vi "Create Device Tree.vi"(8 "error in (no error)":errorcluster caption="错误输入（无错误）", 9 "Item Indent":i16 caption="项缩进", 10 "Tree Control Ref":refnum<vi> caption="树形控件引用", 11 "Project Item Array":refnum<vi>[](array[refnum]) caption="项目项集合") -> (0 "error out":errorcluster caption="错误输出")   [LabVIEW 2013]
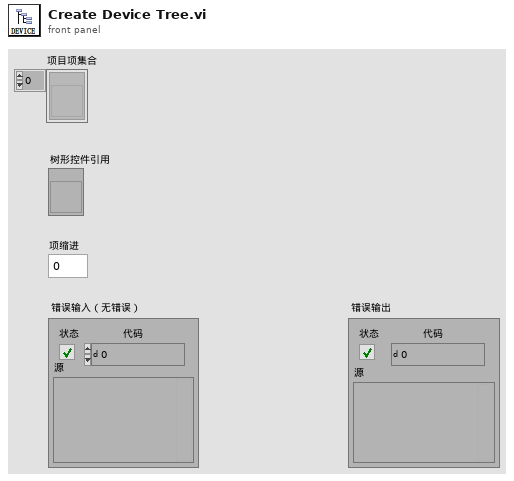
[diagram p1: front panel]
types:
  T1 = cluster{"Left Cell String":string, "Child Text":string[], "Child Tag":string, "Item Indent":i32, "Child Only?":bool, "Glyph Index":i32}
  T2 = typedef "imagedata.ctl" = cluster{"image type":i32, "image depth":i32, "image":u8[], "mask":u8[], "colors":u32[], "Rectangle":cluster{"left":i16, "top":i16, "right":i16, "bottom":i16}}
  T3 = cluster{"Left Cell String":string, "Child Text":string[], "Child Tag":string, "Item Indent":i32, "Child Only?":bool, "Glyph Index":i32}[]
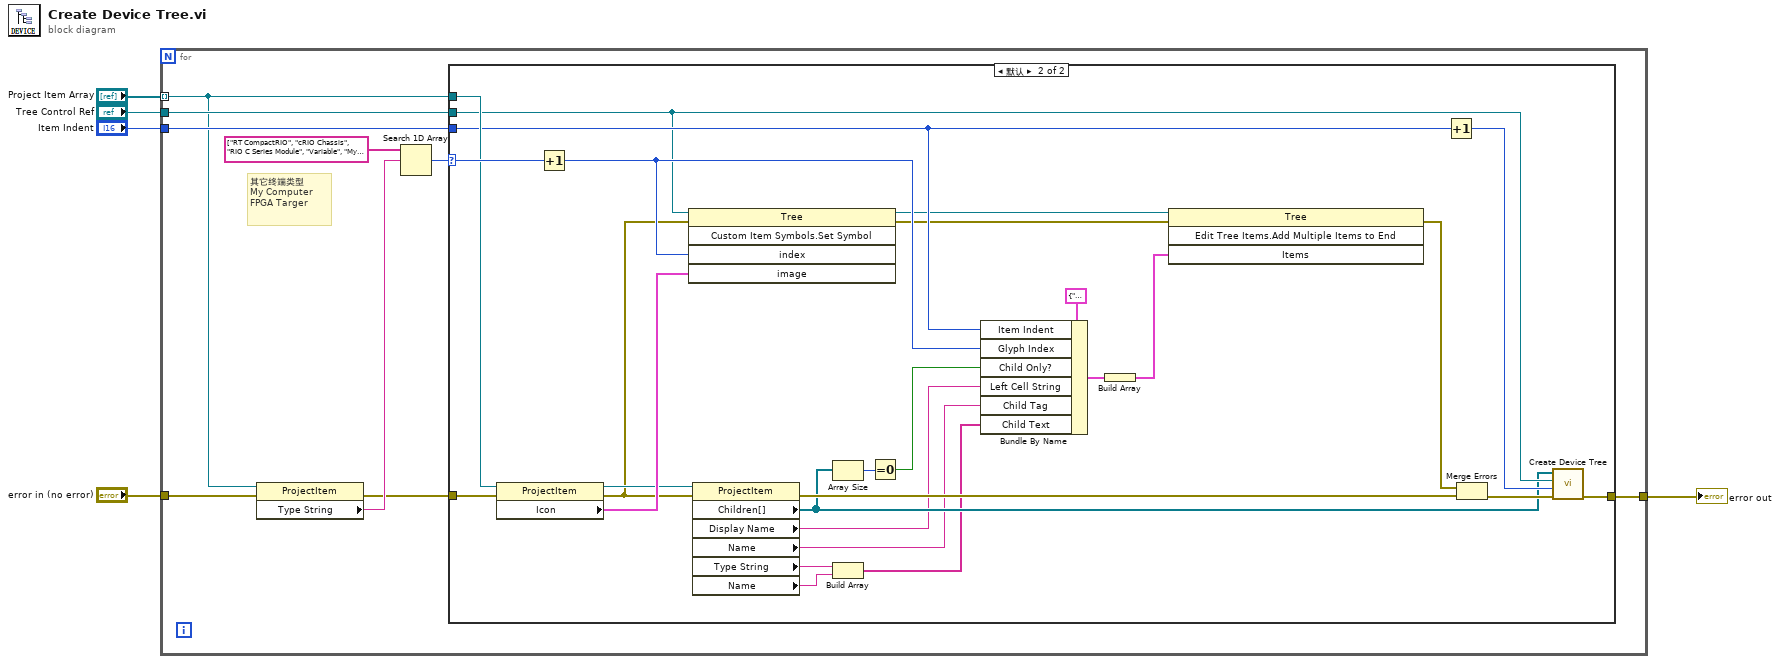
[diagram p0: block diagram]
diagram:
  n1 = for {
    tunnel: "Project Item Array" -> [w7] mode=indexing
    tunnel: "error in (no error)" -> [w6]
    tunnel: "Item Indent" -> [w10]
    tunnel: "Tree Control Ref" -> [w9]
    tunnel: [w8] -> w1
    # "其它终端类型\nMy Computer\nFPGA Targer"
    n2 = property class="ProjectItem"(reference=w7, error in=w6) -> (error out=w11:errorcluster, "Type String"=w13:string)  [unwired: 1 out]
    n3 = Search 1D Array(1D array=string[] ["RT CompactRIO", "cRIO Chassis", "RIO C Series Module", "Variable", "My Computer"], element=w13) -> (index of element=w12:i32)  [unwired: 1 in]
    n4 = case shown="默认" w12 {
      selector: w12 -> [_ w40]
      tunnel: w7 -> [_ w39]
      tunnel: w11 -> [w15 w36]
      tunnel: w10 -> [_ w33]
      tunnel: w9 -> [_ w27]
      tunnel: [w15 w42] -> w8
      frame -1 {
      }
      frame Default {
        n5 = property class="ProjectItem"(reference=w39, error in=w36) -> (reference out=w31:refnum<vi>, error out=w26:errorcluster, "Icon"=w41:T2)
        n6 = Increment(x=w40) -> (x+1=w32:i32)
        n7 = invoke class="Tree" method="Custom Item Symbols.Set Symbol"(reference=w27, error in=w26, "index"=w32, "image"=w41) -> (reference out=w29:refnum<vi>, error out=w28:errorcluster)  [unwired: 1 in, 3 out]
        n8 = property class="ProjectItem"(reference=w31, error in=w26) -> (error out=w30:errorcluster, "Children[]"=w21:refnum<vi>[], "Display Name"=w18:string, "Name"=w20:string, "Type String"=w25:string, "Name"=w24:string)  [unwired: 1 out]
        n9 = Array Size(array=w21) -> (size(s)=w23:i32)
        n10 = Build Array(w25, w24) -> (w19:string[])
        n11 = Equal To 0?(x=w23) -> (x = 0?=w22:bool)
        n12 = Bundle By Name(cluster=T1 {"Left Cell String"="", "Child Text"=[], "Child Tag"="", "Item Indent"=0, "Child Only?"=FALSE, "Glyph Index"=0} ("Item"), "Item Indent"=w33, "Glyph Index"=w32, "Child Only?"=w22, "Left Cell String"=w18, "Child Tag"=w20, "Child Text"=w19) -> (w17:T1)
        n13 = Build Array(w17) -> (w16:T3)
        n14 = invoke class="Tree" method="Edit Tree Items.Add Multiple Items to End"(reference=w29, error in=w28, "Items"=w16) -> (error out=w35:errorcluster)  [unwired: 1 in, 3 out]
        n15 = Increment(x=w33) -> (x+1=w37:i16)
        n16 = Merge Errors(w35, w30) -> (w34:errorcluster)
        n17 = call "Create Device Tree.vi"("error in (no error)"=w34, "Item Indent"=w37, "Tree Control Ref"=w27, "Project Item Array"=w21) -> ("error out"=w42:errorcluster)  [unwired: 7 in]
      }
    }
  }
  "error out" <- w1
